vi "_StopSignal-Core-StopAll.vi"(6 "LIBNAME":string, 8 "error in (no error)":errorcluster, 9 "timeout(ms)":u32=5000, 10 "reason(\"\")":string, 11 "name(\"\")":string[](array[string])) -> (0 "error out":errorcluster, 1 "cache":T1)   [LabVIEW 2019, in "StopSignal.lvlib"]
uses:
  StopSignal.lvlib
  Typedef/StopSignal.ctl
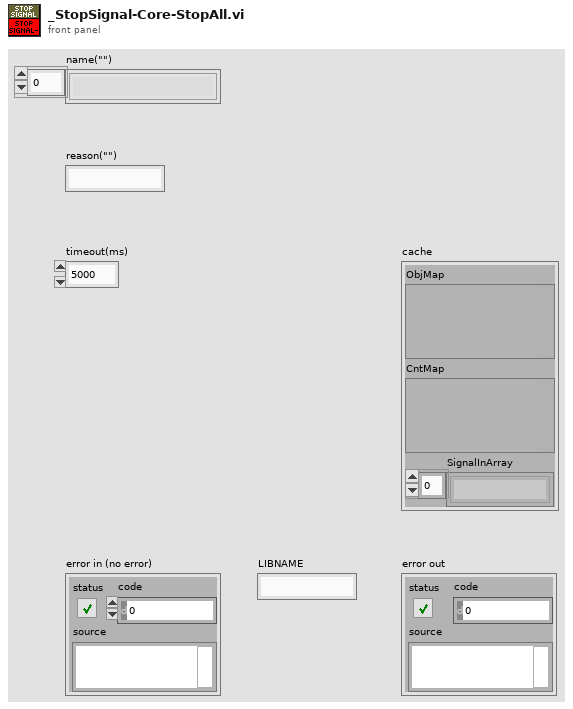
[diagram p1: front panel]
types:
  T1 = cluster{"ObjMap":variant, "CntMap":variant, "SignalInArray":string[]}
  T2 = typedef "StopSignal.lvlib/StopSignal.ctl" = refnum<k1>
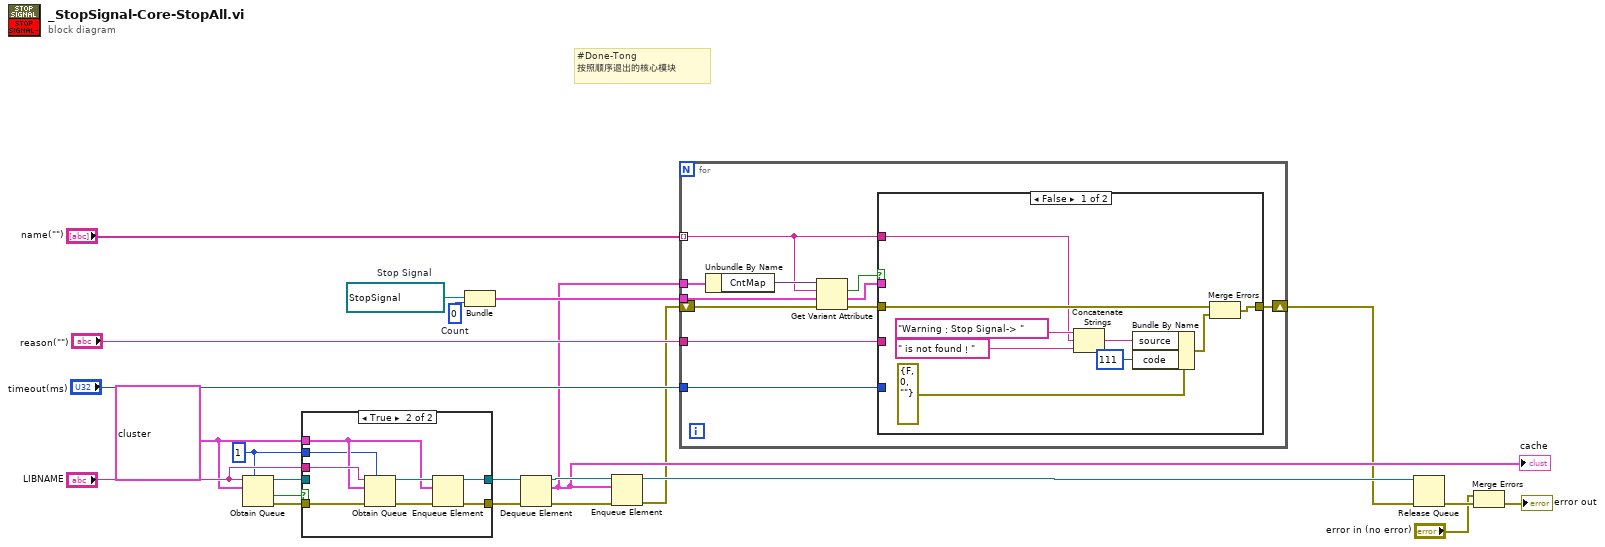
[diagram p0: block diagram]
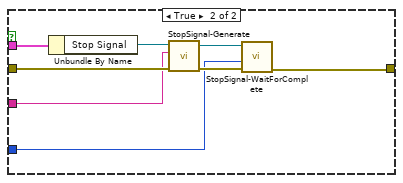
[diagram p2: hidden frame]
diagram:
  w5 = T1 {"ObjMap"=variant, "CntMap"=variant, "SignalInArray"=[]}
  w9 = T2 refnum items=["StopSignal"]  # Stop Signal
  w10 = 0  # Count
  w12 = 1 ("max queue size (-1, unlimited)")
  # "#Done-Tong\n按照顺序退出的核心模块"
  n1 = Obtain Queue(max queue size (-1, unlimited)=w12, name (unnamed)="LIBNAME", element data type=w5) -> (queue out=w20:refnum<queue>, created new?=w22:bool, error out=w21:errorcluster)  [unwired: 2 in]
  n2 = case shown="True" w22 {
    tunnel: w21 -> [w24 w31]
    tunnel: w20 -> [w25 _]
    tunnel: w5 -> [_ w27]
    tunnel: [w24 w33] -> w19
    tunnel: [w25 w32] -> w18
    tunnel: "LIBNAME" -> [_ w28]
    tunnel: w12 -> [_ w26]
    frame False {
    }
    frame True {
      n3 = Obtain Queue(max queue size (-1, unlimited)=w26, name (unnamed)=w28, element data type=w27, error in (no error)=w31) -> (queue out=w29:refnum<queue>, error out=w30:errorcluster)  [unwired: 1 in, 1 out]
      n4 = Enqueue Element(queue=w29, element=w27, error in (no error)=w30) -> (queue out=w32:refnum<queue>, error out=w33:errorcluster)  [unwired: 1 in, 1 out]
    }
  }
  n5 = Bundle("Stop Signal"=w9, "Count"=w10) -> (w8:cluster{"Stop Signal":T2, "Count":i32})  [unwired: 1 in]
  n6 = Dequeue Element(queue=w18, error in (no error)=w19) -> (queue out=w17:refnum<queue>, element=w4:T1, error out=w3:errorcluster)  [unwired: 1 in, 1 out]
  "cache" <- w4
  n7 = Enqueue Element(queue=w17, element=w4, error in (no error)=w3) -> (queue out=w16:refnum<queue>, error out=w2:errorcluster)  [unwired: 1 in, 1 out]
  n8 = for {
    tunnel: "name(\"\")" -> [w39] mode=indexing
    shift-right: [w37] -> w1
    shift-left: w2 -> [w43]
    tunnel: w8 -> [w42]
    tunnel: "reason(\"\")" -> [w36]
    tunnel: "timeout(ms)" -> [w35]
    tunnel: w4 -> [w34]
    n9 = Unbundle By Name(w34) -> ("CntMap"=w44:variant)
    n10 = Get Variant Attribute(Variant=w44, name=w39, default value (empty Variant)=w42, error in=w43) -> (found=w41:bool, value=w40:cluster{"Stop Signal":T2, "Count":i32}, error out=w38:errorcluster)  [unwired: 1 out]
    n11 = case shown="False" w41 {
      tunnel: w40 -> [_ w61]
      tunnel: w39 -> [w51 _]
      tunnel: w38 -> [w53 w59]
      tunnel: [w46 w54] -> w37
      tunnel: w36 -> [_ w58]
      tunnel: w35 -> [_ w55]
      frame False {
        n12 = Concatenate Strings("Warning：Stop Signal-> ", w51, " is not found！") -> (w48:string)
        n13 = Bundle By Name(cluster=errorcluster {"status"=FALSE, "code"=0, "source"=""} ("error constant"), "source"=w48, "code"=111) -> (w45:errorcluster)
        n14 = Merge Errors(w53, w45) -> (w46:errorcluster)
      }
      frame True {
        n15 = Unbundle By Name(w61) -> ("Stop Signal"=w60:T2)
        n16 = call "StopSignal-Generate.vi"("error in (no error)"=w59, "reason(\"\")"=w58, "StopSignal"=w60) -> ("error out"=w56:errorcluster, "StopSignal(dup)"=w57:T2)  [unwired: 7 in]
        n17 = call "StopSignal-WaitForComplete.vi"("error in"=w56, "timeout(ms)"=w55, "StopSignal"=w57) -> ("error out"=w54:errorcluster)  [unwired: 7 in, 1 out]
      }
    }
  }
  n18 = Release Queue(queue=w16, error in (no error)=w1) -> (error out=w23:errorcluster)  [unwired: 1 in, 2 out]
  n19 = Merge Errors("error in (no error)", w23) -> (→"error out":errorcluster)
